vi "ADC.vi"() -> ()   [LabVIEW 2023]
panel:
  out "Output":dbl
  in  "Stop":bool
  in  "Ressolution (bits)":u16
  in  "Maximum Voltage":dbl
  in  "Minimum Voltage":dbl
  in  "Analog Data":dbl
  # "Instructuions:\n1. Enter the obtained analog data \n    from the instrument.\n2. Input the minimum vaue on \n   the scale of the instrument.\n3. Enter ha maximum value on \n   the scale on the maximum.\n4. Enter the resolution bits of the \n   converter present.\n5. press stop to exit the application."
  # "Note:\n- The minimum voltage should always \n    be less than the maximum voltage\n- The analog data should be within the\n   range of the maximum and the \n   minimum voltage.\n- In case of invalid inputs, the output \n   will result in -1.."
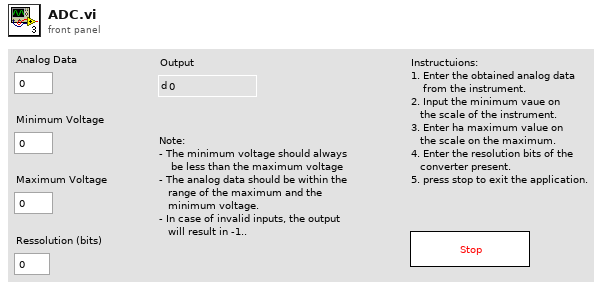
[diagram p1: front panel]
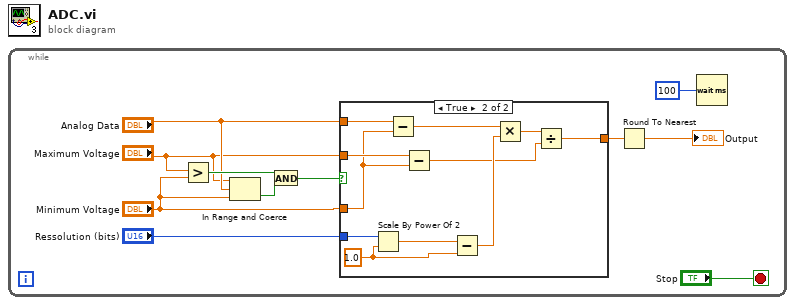
[diagram p0: block diagram]
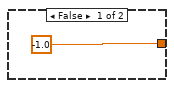
[diagram p2: hidden frame]
diagram:
  n1 = while {
    stop <- "Stop" stop-if-true
    n2 = Greater?(x="Maximum Voltage", y="Minimum Voltage") -> (0:w7:bool)
    n3 = In Range and Coerce(upper limit="Maximum Voltage", x="Analog Data", lower limit="Minimum Voltage") -> (In Range?=w2:bool)  [unwired: 1 out]
    n4 = And(x=w7, y=w2) -> (x .and. y?=w6:bool)
    n5 = case shown="True" w6 {
      tunnel: "Maximum Voltage" -> [_ w23]
      tunnel: "Analog Data" -> [_ w22]
      tunnel: "Minimum Voltage" -> [_ w21]
      tunnel: [-1.0 w16] -> w10
      tunnel: "Ressolution (bits)" -> [_ w14]
      frame False {
      }
      frame True {
        w13 = 1.0
        n6 = Scale By Power Of 2(n=w14, x=w13) -> (x*2^n=w20:dbl)
        n7 = Subtract(x=w22, y=w21) -> (x-y=w19:dbl)
        n8 = Subtract(x=w23, y=w21) -> (x-y=w17:dbl)
        n9 = Subtract(x=w20, y=w13) -> (x-y=w18:dbl)
        n10 = Multiply(x=w19, y=w18) -> (x*y=w15:dbl)
        n11 = Divide(x=w15, y=w17) -> (x/y=w16:dbl)
      }
    }
    n12 = Round To Nearest(number=w10) -> (nearest integer value=→"Output":dbl)
    n13 = Wait (ms)(milliseconds to wait=u32 100) -> ()  [unwired: 1 out]
  }
